vi "SingleAcquisitionExpRes.vi"() -> ()   [LabVIEW 2018]
uses:
  D:/SVN/PM/sdk/AppSamples/LabVIEWSamples/trunk/Release/2018/Dependencies/PVCamNET.dll
  Dependencies/PVCamNET.dll
panel:
  out "Exposure Resolution":string
  in  "?":bool
  in  "Exposure time":dbl=30.0
  in  "?":bool
  # "SingleAcquisitionExpRes.vi\n\nDescription:\nThis sample code lets the user use single acqusition mode\nwith the user's preferred exposure resolution type. \n\nSteps to run:\n\n0. Before running the VI go to Window and update the Exposure Resolution index\n1. Click \"Run\"\n2. Enter exposure time\n3. Click \"START\"\n4. Click \"STOP\""
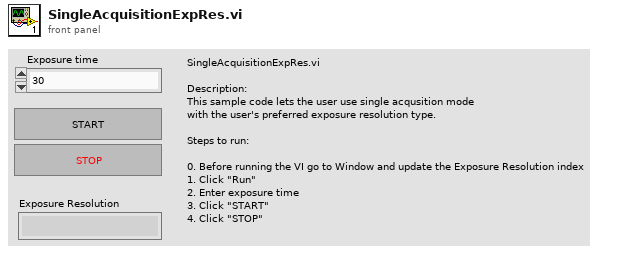
[diagram p1: front panel]
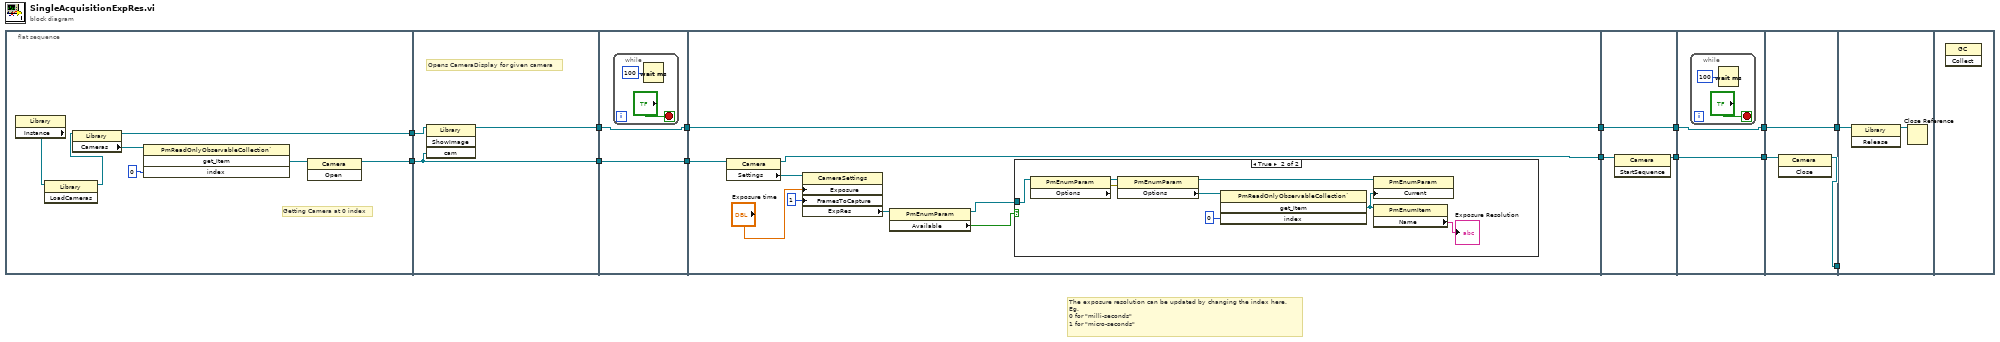
[diagram p0: block diagram]
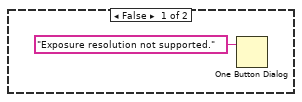
[diagram p2: hidden frame]
diagram:
  # "The exposure resolution can be updated by changing the index here.\nEg. \n0 for \"milli-seconds\"\n1 for \"micro-seconds\""
  n1 = flat-sequence {
    tunnel: [w17] -> w14
    tunnel: [w18] -> w13
    tunnel: w14 -> [w24]
    tunnel: w13 -> [w23]
    tunnel: [w23] -> w12
    tunnel: [w22] -> w11
    tunnel: w12 -> [w26]
    tunnel: [w26] -> w9
    tunnel: w11 -> [w25]
    tunnel: [w25] -> w10
    tunnel: [w37] -> w8
    tunnel: [w36] -> w7
    tunnel: w10 -> [w36]
    tunnel: w9 -> [w35]
    tunnel: w8 -> [w48]
    tunnel: [w47] -> w6
    tunnel: [w49] -> w5
    tunnel: w7 -> [w49]
    tunnel: w6 -> [w51]
    tunnel: [w51] -> w2
    tunnel: [w50] -> w1
    tunnel: w5 -> [w50]
    tunnel: w2 -> [w56]
    tunnel: w1 -> [w54]
    tunnel: [w55] -> w4
    tunnel: [w54] -> w3
    tunnel: w4 -> [_]
    tunnel: w3 -> [w58]
    frame #0 {
      # "Getting Camera at 0 index"
      n2 = property class="Library"() -> ("Instance"=w16:refnum<k24>)  [unwired: 2 in, 2 out]
      n3 = invoke class="Library" method="LoadCameras"(reference=w16) -> (reference out=w15:refnum<k24>)  [unwired: 2 in, 2 out]
      n4 = property class="Library"(reference=w15) -> (reference out=w17:refnum<k24>, "Cameras"=w21:refnum<k24>)  [unwired: 1 in, 1 out]
      n5 = invoke class="PmReadOnlyObservableCollection`" method="get_Item"(reference=w21, "index"=0) -> ("get_Item"=w19:refnum<k24>)  [unwired: 2 in, 3 out]
      n6 = invoke class="Camera" method="Open"(reference=w19) -> (reference out=w18:refnum<k24>)  [unwired: 2 in, 2 out]
    }
    frame #1 {
      # "Opens CameraDisplay for given camera"
      n7 = invoke class="Library" method="ShowImage"(reference=w24, "cam"=w23) -> (reference out=w22:refnum<k24>)  [unwired: 2 in, 3 out]
    }
    frame #2 {
      n8 = while {
        stop <- "?" stop-if-true
        n9 = Wait (ms)(milliseconds to wait=u32 100) -> ()  [unwired: 1 out]
      }
    }
    frame #3 {
      n10 = property class="Camera"(reference=w35) -> (reference out=w37:refnum<k24>, "Settings"=w33:refnum<k24>)  [unwired: 1 in, 1 out]
      n11 = property class="CameraSettings"(reference=w33, "Exposure"="Exposure time", "FramesToCapture"=u16 1) -> ("ExpRes"=w31:refnum<k24>)  [unwired: 1 in, 2 out]
      n12 = property class="PmEnumParam"(reference=w31) -> (reference out=w29:refnum<k24>, "Available"=w30:bool)  [unwired: 1 in, 1 out]
      n13 = case shown="True" w30 {
        tunnel: w29 -> [_ w46]
        frame False {
          n14 = One Button Dialog(message="Exposure resolution not supported.") -> ()  [unwired: 1 in, 1 out]
        }
        frame True {
          n15 = property class="PmEnumParam" props=["Options"](reference=w46) -> (reference out=w44:refnum<k24>, error out=w45:errorcluster)  [unwired: 1 in, 1 out]
          n16 = property class="PmEnumParam"(reference=w44, error in=w45) -> (reference out=w41:refnum<k24>, "Options"=w43:refnum<k24>)  [unwired: 1 out]
          n17 = invoke class="PmReadOnlyObservableCollection`" method="get_Item"(reference=w43, "index"=0) -> ("get_Item"=w40:refnum<k24>)  [unwired: 2 in, 3 out]
          n18 = property class="PmEnumParam"(reference=w41, "Current"=w40) -> ()  [unwired: 1 in, 2 out]
          n19 = property class="PmEnumItem"(reference=w40) -> ("Name"=→"Exposure Resolution":string)  [unwired: 1 in, 2 out]
        }
      }
    }
    frame #4 {
      n20 = invoke class="Camera" method="StartSequence"(reference=w48) -> (reference out=w47:refnum<k24>)  [unwired: 2 in, 2 out]
    }
    frame #5 {
      n21 = while {
        stop <- "?" stop-if-true
        n22 = Wait (ms)(milliseconds to wait=u32 100) -> ()  [unwired: 1 out]
      }
    }
    frame #6 {
      n23 = invoke class="Camera" method="Close"(reference=w56) -> (reference out=w55:refnum<k24>)  [unwired: 2 in, 2 out]
    }
    frame #7 {
      n24 = invoke class="Library" method="Release"(reference=w58) -> (reference out=w57:refnum<k24>)  [unwired: 2 in, 2 out]
      n25 = Close Reference(reference=w57) -> ()  [unwired: 1 in, 1 out]
    }
    frame #8 {
      n26 = invoke class="GC" method="Collect"() -> ()  [unwired: 3 in, 3 out]
    }
  }
